vi "Array Manipulation.vi"() -> ()   [LabVIEW 2012]
doc: "本VI演示了不同的处理数据的数组函数。也有范例演示了如何使用LabVIEW内置的多态功能便捷地修改数组中的数据。\n\n检查不同分支，读取程序框图中的说明以了解更多信息。"
uses:
  <vilib>/measure/NI_MABase.lvlib
panel:
  in  "停止按钮":bool
  in  "选项卡控件":T1(tab)
  out "连接的数据数组":dbl[](array[numeric])
  out "连接的数据":dbl[](graph)
  in  "减？":bool
  out "加/减数据数组":dbl[](array[numeric])
  out "加/减数据":dbl[](graph)
  in  "选择通道":u16(ring) items=["通道0", "通道1"]
  out "数据数组的单通道":dbl[](array[numeric])
  out "数据的单通道":dbl[](graph)
  out "数组大小":i32
  in  "偏移量":dbl(slide)=-8.326672684688674e-17 scale=-5.0..5.0
  out "波形数据":waveform(dbl)[](graph)
  out "数据通道数组":dbl[][](array[numeric])
  in  "通道1偏置":dbl(slide)=-8.326672684688674e-17 scale=-5.0..5.0
  out "全部数据通道":dbl[][](graph)
  out "数组大小":i32[](array[numeric])
  out "子集数据数组":dbl[][](array[numeric])
  in  "开始值":i32(slide)=10 scale=0.0..1000.0
  out "子集数据":dbl[][](graph)
  in  "长度":i32(slide)=1000 scale=0.0..1000.0
  # "行"
  # "列"
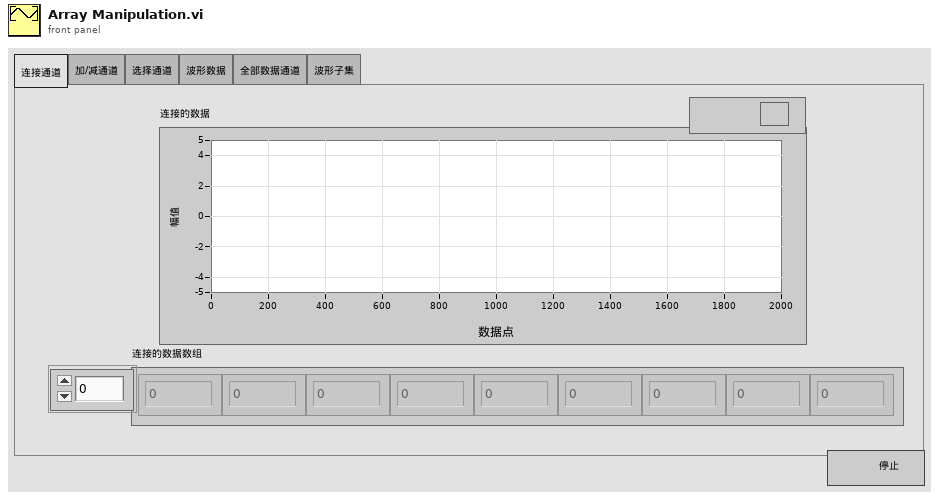
[diagram p1: front panel]
types:
  T1 = enum32{"连接通道", "加/减通道", "选择通道", "波形数据", "全部数据通道", "波形子集"}
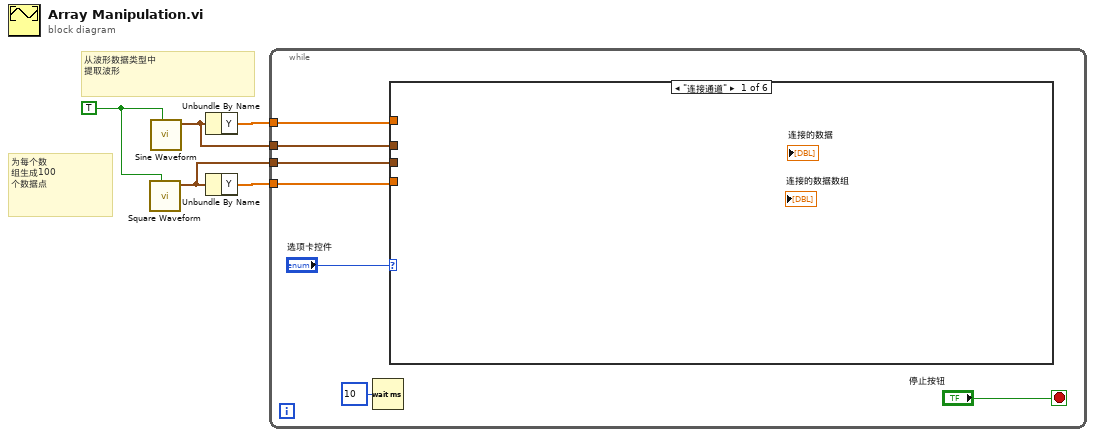
[diagram p0: block diagram]
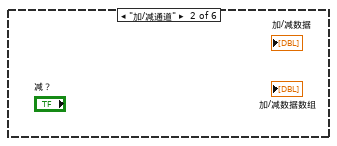
[diagram p2: hidden frame]
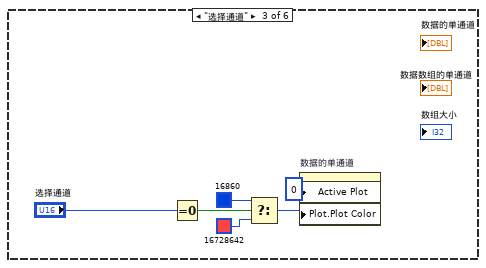
[diagram p3: hidden frame]
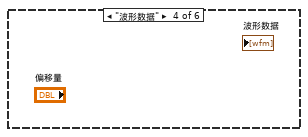
[diagram p4: hidden frame]
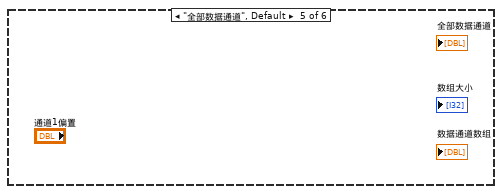
[diagram p5: hidden frame]
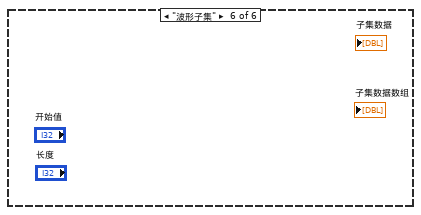
[diagram p6: hidden frame]
diagram:
  w5 = TRUE
  # "从波形数据类型中\n提取波形"
  # "为每个数\n组生成100\n个数据点"
  n1 = call <vilib>:"Square Waveform.vi"("reset signal"=w5) -> ("signal out"=w1:waveform(dbl))  [unwired: 9 in, 1 out]
  n2 = call <vilib>:"Sine Waveform.vi"("reset signal"=w5) -> ("signal out"=w2:waveform(dbl))  [unwired: 9 in, 1 out]
  n3 = Unbundle By Name ("获取波形成分")(w2) -> ("Y"=w4:dbl[])
  n4 = Unbundle By Name ("获取波形成分")(w1) -> ("Y"=w3:dbl[])
  n5 = while {
    tunnel: w4 -> [w10]
    tunnel: w3 -> [w9]
    tunnel: w2 -> [w8]
    tunnel: w1 -> [w7]
    stop <- "停止按钮" stop-if-true
    n6 = Wait (ms) ("等待(ms)")(milliseconds to wait=u32 10 ("等待时间（毫秒）")) -> ()  [unwired: 1 out]
    n7 = case shown="\"连接通道\"" "选项卡控件" {
      tunnel: w10 -> [_ _ _ _ _ _]
      tunnel: w9 -> [_ _ _ _ _ _]
      tunnel: w8 -> [_ _ _ _ _ _]
      tunnel: w7 -> [_ _ _ _ _ _]
      frame "连接通道" {
      }
      frame "加/减通道" {
      }
      frame "选择通道" {
        n8 = Equal To 0? ("等于0？")(x="选择通道") -> (x = 0?=w14:bool)
        n9 = Select ("选择")(t=u32 16860, s=w14, f=u32 16728642) -> (s? t:f=w17:u32)
        n10 = property on="数据的单通道" class="WFGraph (严格)"("Active Plot"=u32 0 ("活动曲线"), "Plot.Plot Color"=w17) -> ()  [unwired: 2 in, 2 out]
      }
      frame "波形数据" {
      }
      frame "全部数据通道", Default {
      }
      frame "波形子集" {
      }
    }
  }
